vi "Computer_Board.vi"() -> (0 "Array":dbl[][](array[numeric]))   [LabVIEW 2026]
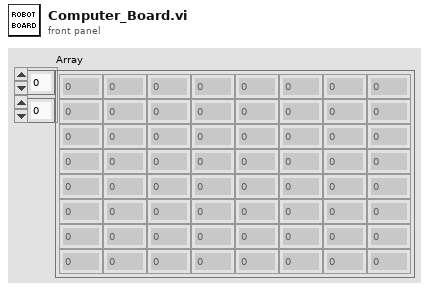
[diagram p1: front panel]
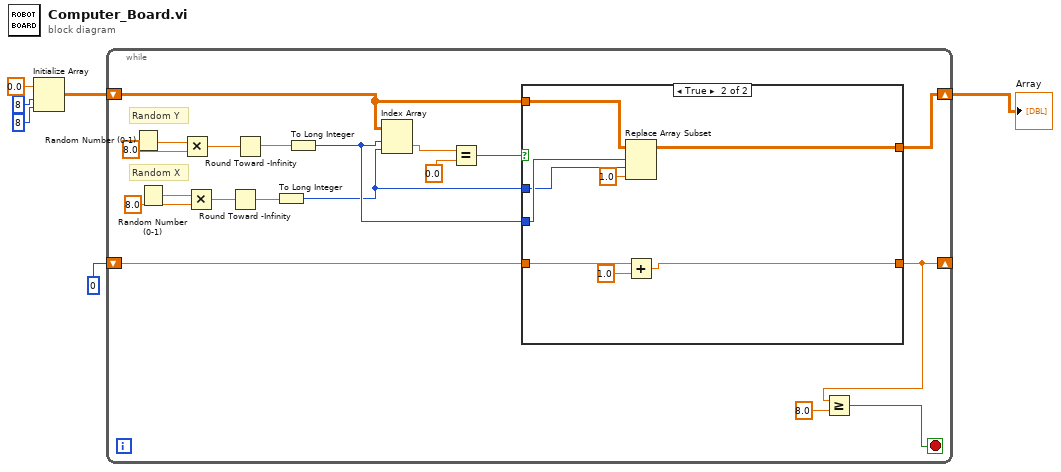
[diagram p0: block diagram]
diagram:
  n1 = Initialize Array(0.0 ("element"), 8 ("dimension size"), 8 ("dimension size")) -> (w3:dbl[][])
  n2 = while {
    shift-right: [w11] -> w1
    shift-left: w3 -> [w14]
    shift-right: [w9] -> _
    shift-left: 0 -> [w10]
    stop <- w7 stop-if-true
    # "Random Y"
    # "Random X"
    n3 = Random Number (0-1)() -> (number: 0 to 1=w25:dbl)
    n4 = Random Number (0-1)() -> (number: 0 to 1=w23:dbl)
    n5 = Multiply(x=w25, y=8.0) -> (x*y=w21:dbl)
    n6 = Multiply(x=w23, y=8.0) -> (x*y=w20:dbl)
    n7 = Round Toward -Infinity(1:w20) -> (0:w18:dbl)
    n8 = Round Toward -Infinity(1:w21) -> (0:w19:dbl)
    n9 = To Long Integer(number=w18) -> (32bit integer=w12:i32)
    n10 = To Long Integer(number=w19) -> (32bit integer=w13:i32)
    n11 = Index Array(array=w14, index (row)=w13, index (col)=w12) -> (element=w17:dbl)
    n12 = Equal?(x=w17, y=0.0) -> (x = y?=w15:bool)
    n13 = case shown="True" w15 {
      tunnel: w14 -> [w26 w35]
      tunnel: w13 -> [_ w34]
      tunnel: w12 -> [_ w33]
      tunnel: [w26 w31] -> w11
      tunnel: w10 -> [w27 w29]
      tunnel: [w27 w28] -> w9
      frame False {
      }
      frame True {
        n14 = Replace Array Subset(array=w35, new element=1.0 ("new element/subarray"), index (row)=w34, index (col)=w33) -> (w31:dbl[][])
        n15 = Add(x=w29, y=1.0) -> (x+y=w28:dbl)
      }
    }
    n16 = Greater Or Equal?(x=w9, y=8.0) -> (x >= y?=w7:bool)
  }
  "Array" <- w1
